vi "Kinesis - KLSnnn - Set Power.vi"() -> ()   [LabVIEW 2012]
uses:
  U:/Kinesis LabVIEW Website Examples/Thorlabs.MotionControl.Controls.dll
  Thorlabs.MotionControl.Controls.dll
  U:/Kinesis LabVIEW Website Examples/ThorLabs.MotionControl.KCube.LaserSourceCLI.dll
  ThorLabs.MotionControl.KCube.LaserSourceCLI.dll
panel:
  in  "Serial Number":string
  in  "?":bool
  in  "Power":dbl
  in  "?":bool
  in  "?":bool
  in  "?":bool
  in  "KCubeLaserSourceControl":refnum<k24>(container)
  # "Notes:"
  # "- Ensure that the appropriate .DLLs are copied into your Project Folder. Check that the correct bit type are used depending on your version of LabVIEW\ni.e. 32-bit or 64-bit.\n\n\n\n\n\n\n\n\n\n\n\n\n\n\n- Open the example VI through the LabVIEW Project Explorer to correctly load the User Interface from Thorlabs.MotionControl.Controls.dll."
  # "Thorlabs Hardware: KLS635/KLS1550\nhttps://www.thorlabs.com/newgrouppage9.cfm?objectgroup_id=2922"
  # "Description: This VI will enable you to set the Laser Output On/Off, as well as set the Output Power of the laser source."
  # "Instructions: \n1) Connect your KLSnnn device to your PC & power the device. For full device setup, the device product manual can be found on our website here.\n - https://www.thorlabs.com/newgrouppage9.cfm?objectgroup_id=2922&pn=KLS635\n2)  Set the interlock key to 'ON'\n3) Enter the device serial number below.\n4) Click 'Run' in the LabVIEW Toolbar.\n5) Toggle the Laser ON/OFF with the buttons below.\n6) Enter a Power in mW & click 'SET POWER' to adjust the Laser Output Power.\n5) To end the Program, click 'END'."
  # "LASER ON/OFF"
  # "Example Image of .NET Controller - VI opened via Project Explorer/ not opened via Project Explorer"
  # "VI Not Opened via Project Explorer"
  # "VI Opened via Project Explorer"
  # "- To explore the range of methods available, please visit the .NET API, included with your Kinesis software.\n\n- For tips on building your own VIs with Thorlabs Motion Control Hardware, please see our LabVIEW Guide here.\nhttps://www.thorlabs.com/newgrouppage9.cfm?objectgroup_id=10285"
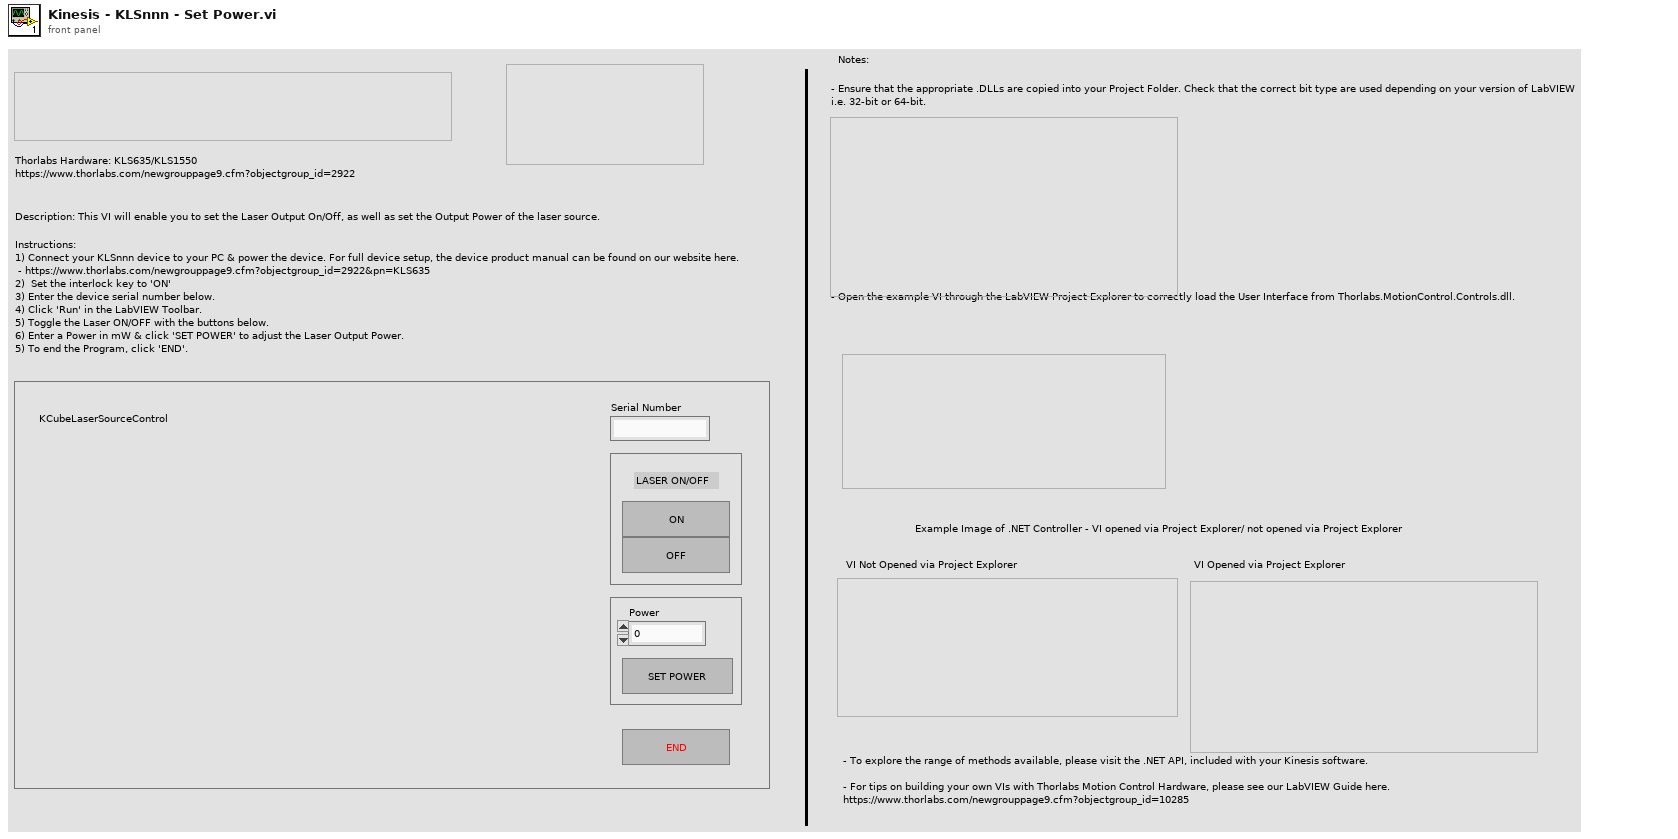
[diagram p1: front panel]
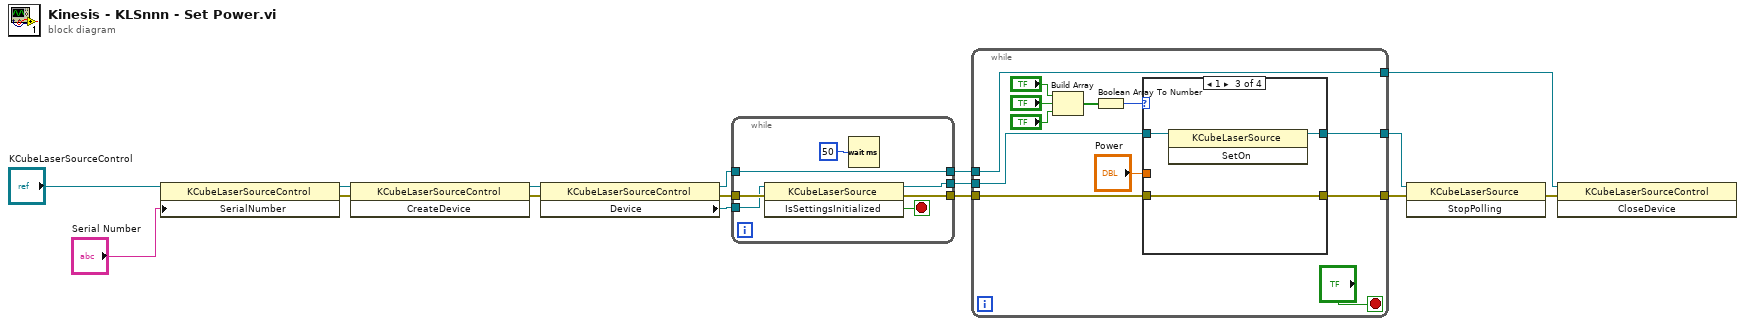
[diagram p0: block diagram]
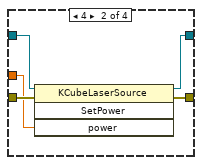
[diagram p3: hidden frame]
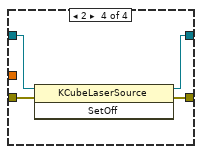
[diagram p4: hidden frame]
diagram:
  n1 = property class="KCubeLaserSourceControl"(reference="KCubeLaserSourceControl", "SerialNumber"="Serial Number") -> (reference out=w15:refnum<k24>, error out=w12:errorcluster)  [unwired: 1 in]
  n2 = invoke class="KCubeLaserSourceControl" method="CreateDevice"(reference=w15, error in=w12) -> (reference out=w14:refnum<k24>, error out=w11:errorcluster)  [unwired: 1 in, 1 out]
  n3 = property class="KCubeLaserSourceControl"(reference=w14, error in=w11) -> (reference out=w4:refnum<k24>, error out=w10:errorcluster, "Device"=w13:refnum<k24>)
  n4 = while {
    tunnel: w13 -> [w18]
    tunnel: [w21] -> w2
    tunnel: w10 -> [w20]
    tunnel: [w19] -> w1
    tunnel: [w17] -> w5
    tunnel: w4 -> [w17]
    stop <- w23 stop-if-true
    n5 = invoke class="KCubeLaserSource" method="IsSettingsInitialized"(reference=w18, error in=w20) -> (reference out=w21:refnum<k24>, error out=w19:errorcluster, "IsSettingsInitialized"=w23:bool)  [unwired: 1 in]
    n6 = Wait (ms)(milliseconds to wait=u32 50) -> ()  [unwired: 1 out]
  }
  n7 = while {
    tunnel: w2 -> [w28]
    tunnel: w1 -> [w33]
    tunnel: [w34] -> w9
    tunnel: [w27] -> w8
    tunnel: [w24] -> w6
    tunnel: w5 -> [w24]
    stop <- "?" stop-if-true
    n8 = Build Array("?", "?", "?") -> (w30:bool[])
    n9 = Boolean Array To Number(Boolean array=w30) -> (number=w29:u32)
    n10 = case shown="1" w29 {
      tunnel: [w36 w39 w45 w46] -> w34
      tunnel: w33 -> [w36 w41 w45 w48]
      tunnel: w28 -> [w37 w42 w44 w49]
      tunnel: [w37 w40 w43 w47] -> w27
      tunnel: "Power" -> [_ w38 _ _]
      frame 0, Default {
      }
      frame 4 {
        n11 = invoke class="KCubeLaserSource" method="SetPower"(reference=w42, error in=w41, "power"=w38) -> (reference out=w40:refnum<k24>, error out=w39:errorcluster)  [unwired: 1 in, 2 out]
      }
      frame 1 {
        n12 = invoke class="KCubeLaserSource" method="SetOn"(reference=w44) -> (reference out=w43:refnum<k24>)  [unwired: 2 in, 2 out]
      }
      frame 2 {
        n13 = invoke class="KCubeLaserSource" method="SetOff"(reference=w49, error in=w48) -> (reference out=w47:refnum<k24>, error out=w46:errorcluster)  [unwired: 1 in, 1 out]
      }
    }
  }
  n14 = invoke class="KCubeLaserSource" method="StopPolling"(reference=w8, error in=w9) -> (error out=w3:errorcluster)  [unwired: 1 in, 2 out]
  n15 = invoke class="KCubeLaserSourceControl" method="CloseDevice"(reference=w6, error in=w3) -> ()  [unwired: 1 in, 3 out]
